vi "Test_output_mixing2.vi"() -> ()   [LabVIEW 2013]
panel:
  out "max value 2":i16
  out "max value":i16
  out "Waveform Graph 3":i16[](graph)
  out "Waveform Graph 2":i16[](graph)
  out "Array 2":i16[](array[numeric])
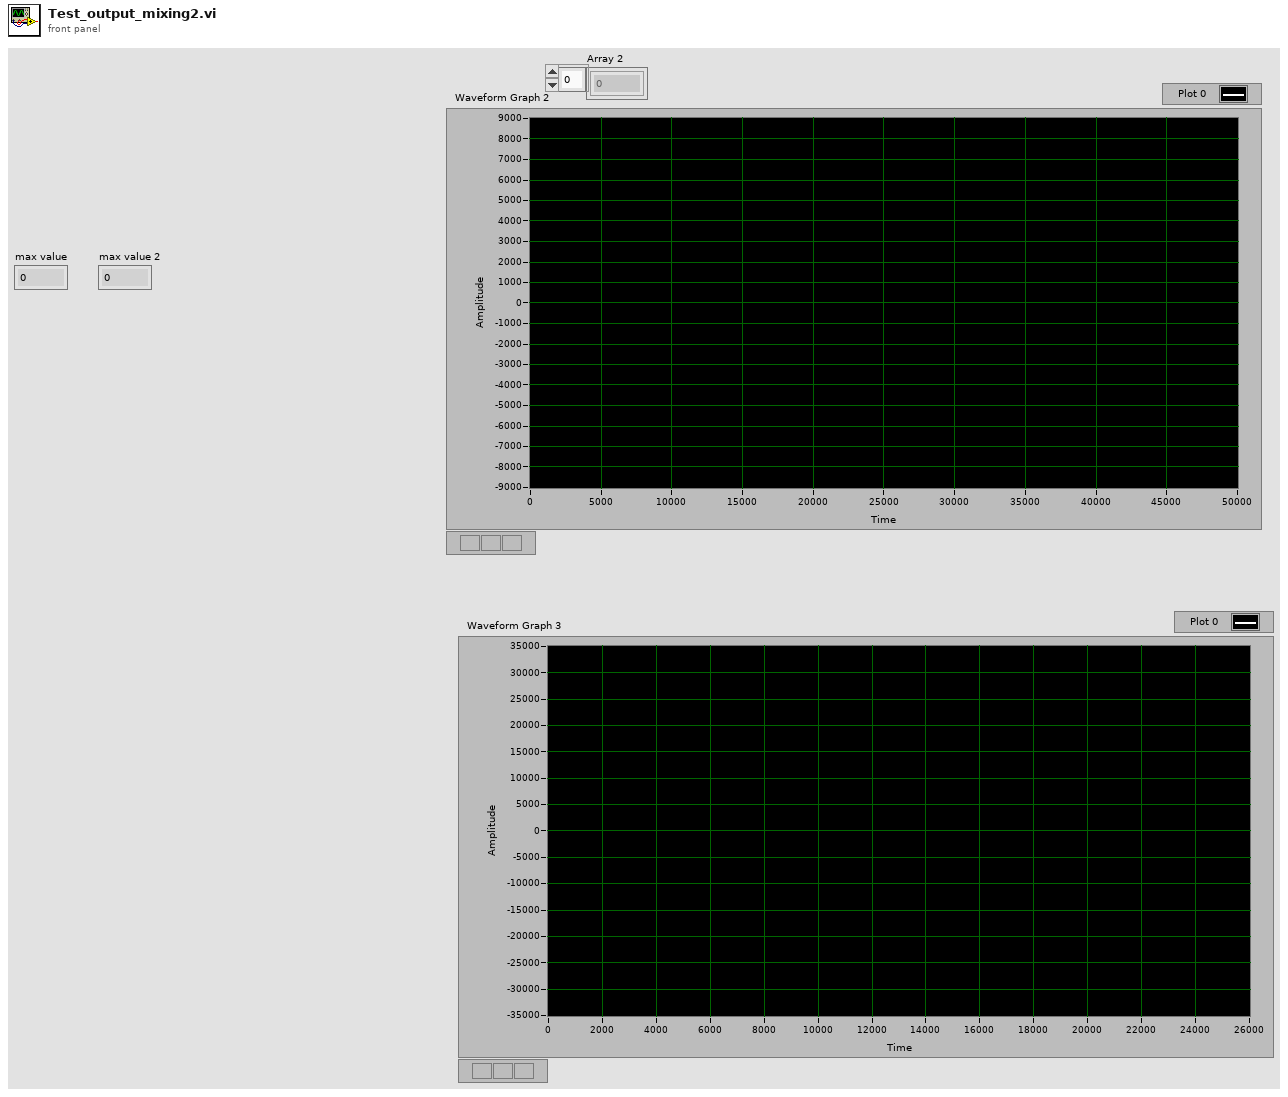
[diagram p1: front panel]
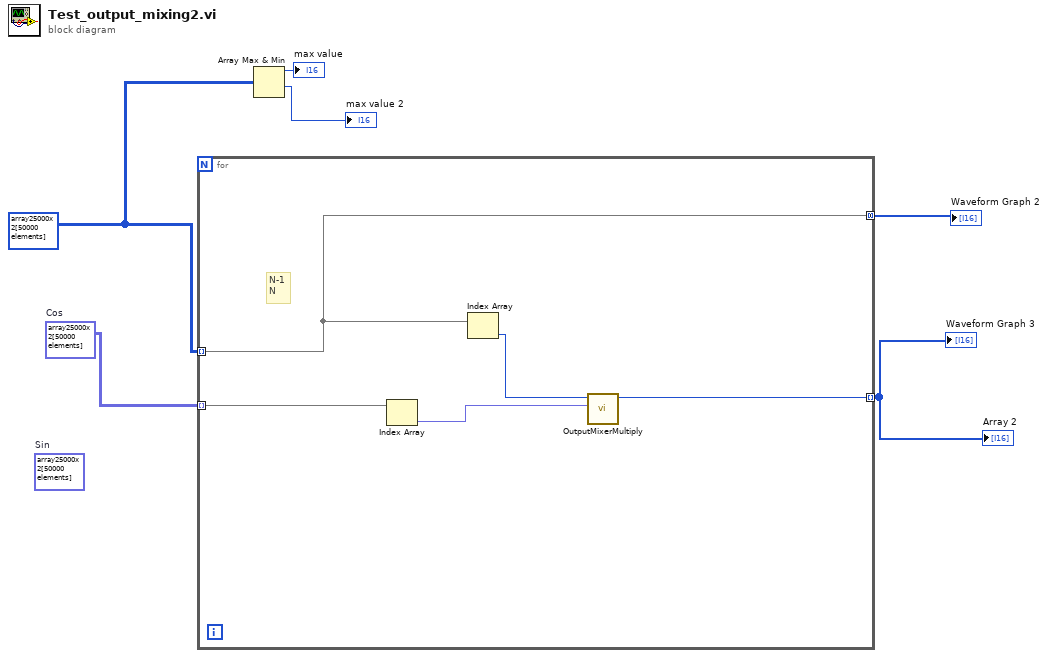
[diagram p0: block diagram]
diagram:
  w1 = i16[][] array25000x2[50000 elements] ("simdata")
  w5 = fxp<+/-,16,0>[][] array25000x2[50000 elements]  # Cos
  (unwired) fxp<+/-,16,0>[][] array25000x2[50000 elements]  # Sin
  n1 = for {
    tunnel: w1 -> [w11] mode=indexing
    tunnel: [w11] -> w6 mode=concatenating
    tunnel: w5 -> [w9] mode=indexing
    tunnel: [w7] -> w4 mode=indexing
    # "N-1\nN"
    n2 = Index Array(array=w9) -> (element=w8:fxp<+/-,16,0>)  [unwired: 1 in]
    n3 = Index Array(array=w11) -> (element=w10:i16)  [unwired: 1 in]
    n4 = call "OutputMixerMultiply.vi"("x"=w8, "y"=w10) -> ("x*y"=w7:i16)  [unwired: 9 in]
  }
  "Array 2" <- w4
  "Waveform Graph 2" <- w6
  "Waveform Graph 3" <- w4
  n5 = Array Max & Min(array=w1) -> (max value=→"max value":i16, min value=→"max value 2":i16)  [unwired: 2 out]
